vi "Check data length.vi"(8 "error in":errorcluster, 11 "# samples in buffer":u16) -> (0 "error out":errorcluster, 2 "Modbus Function":T1, 3 "# samples in buffer out":u16)   [LabVIEW 2017]
uses:
  Ctl/Modbus function.ctl
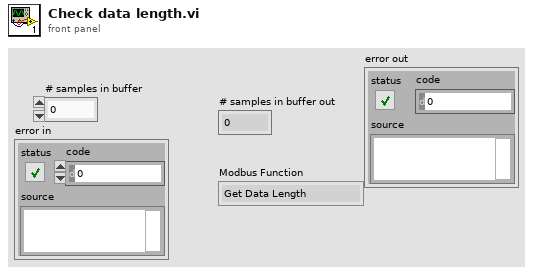
[diagram p1: front panel]
types:
  T1 = typedef "Modbus function.ctl" = enum16{"Get Data Length", "Normal Mode", "Bulk Mode"}
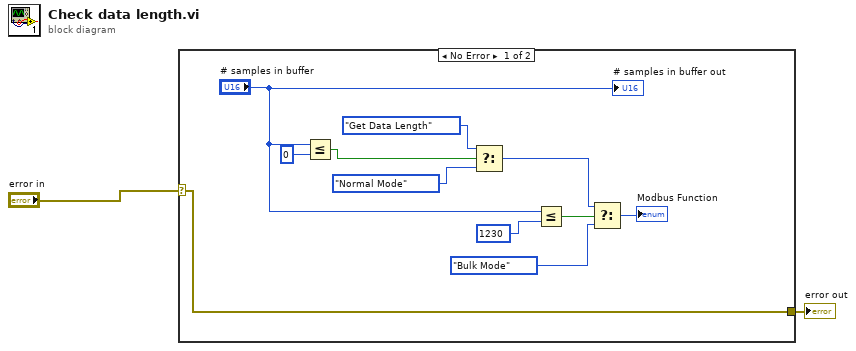
[diagram p0: block diagram]
diagram:
  n1 = case shown="No Error" "error in" {
    selector: "error in" -> [w3 w14]
    tunnel: [w3 w14] -> w1
    frame No Error {
      n2 = Less Or Equal?(x="# samples in buffer", y=u16 0) -> (x <= y?=w12:bool)
      n3 = Select(t=Modbus_function."Get Data Length" ("Modbus"), s=w12, f=Modbus_function."Normal Mode" ("Modbus")) -> (s? t:f=w9:T1)
      n4 = Less Or Equal?(x="# samples in buffer", y=u16 1230) -> (x <= y?=w10:bool)
      n5 = Select(t=w9, s=w10, f=Modbus_function."Bulk Mode" ("Modbus")) -> (s? t:f=→"Modbus Function":T1)
      "# samples in buffer out" <- "# samples in buffer"
    }
    frame Error {
    }
  }
  "error out" <- w1
